vi "LJM logger data file write.vi"(0 "Current Data File In":path, 1 "Write To File":bool, 2 "Currently Writing":bool, 3 "Data File Prefix":string="data", 5 "Working Directory":path, 7 "Log data":string, 9 "Header String":string, 11 "max file size (bytes)":i32=100000000, 15 "Starting #":u32) -> (4 "Current Data File Out":path, 10 "Data File #":u32)   [LabVIEW 2026]
panel:
  out "runtime ms":u32
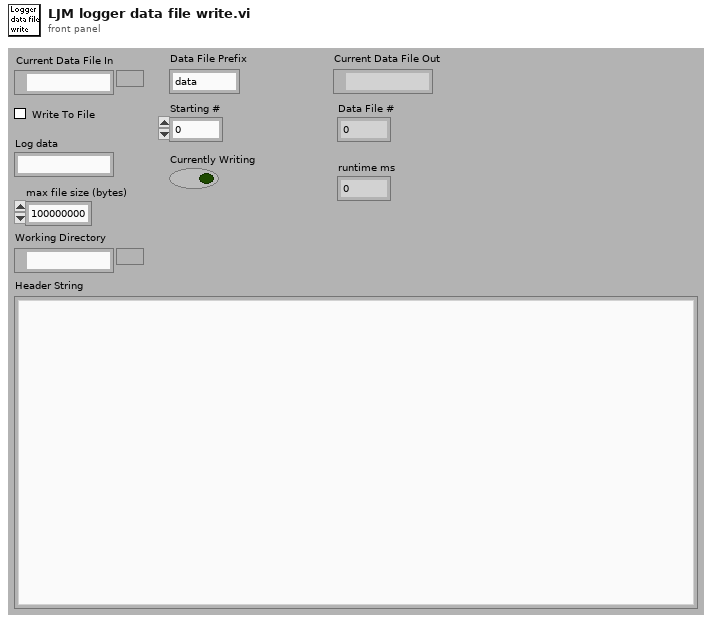
[diagram p1: front panel]
types:
  T1 = enum16{"open", "open or create", "create or replace", "create", "open (read only)"}
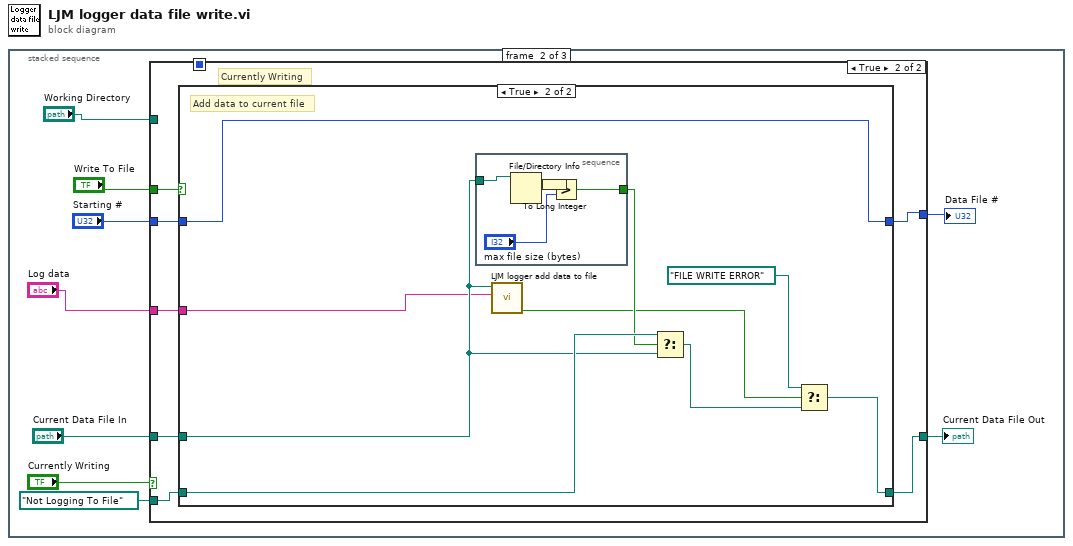
[diagram p0: block diagram]
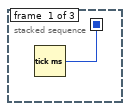
[diagram p2: hidden frame]
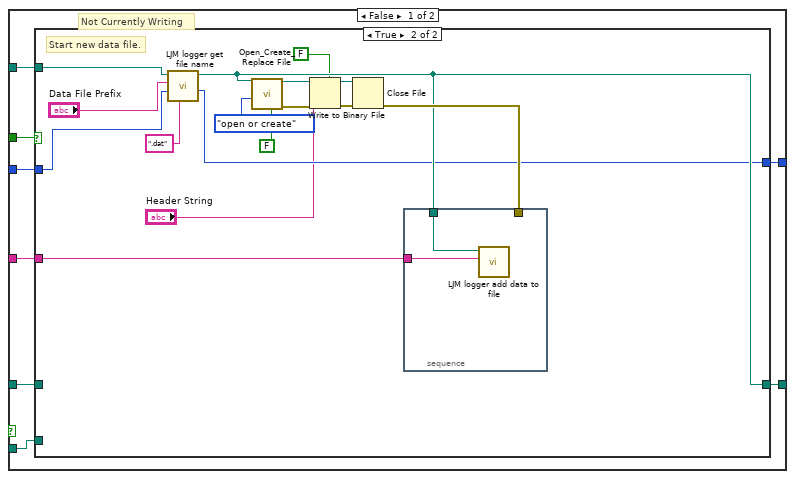
[diagram p3: hidden frame]
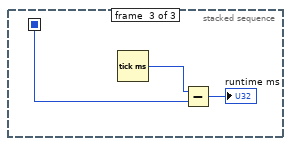
[diagram p6: hidden frame]
diagram:
  n1 = stacked-sequence {
    seq-local: [w1 _ _] -> [_ _ w63]
    frame #0 {
      n2 = Tick Count (ms)() -> (millisecond timer value=w1:u32)
    }
    frame #1 {
      n3 = case shown="True" "Currently Writing" {
        tunnel: "Current Data File In" -> [w18 w45]
        tunnel: "Write To File" -> [w16 w44]
        tunnel: [w17 w42] -> w8
        tunnel: path "Not Logging To File" ("y") -> [w15 w43]
        tunnel: "Starting #" -> [w14 w41]
        tunnel: [w13 w40] -> w5
        tunnel: "Log data" -> [w12 w39]
        tunnel: "Working Directory" -> [w11 _]
        frame False {
          # "Not Currently Writing"
          n4 = case shown="True" w16 {
            tunnel: w18 -> [_ _]
            tunnel: [w20 w28] -> w17
            tunnel: w15 -> [w20 _]
            tunnel: w14 -> [w19 w27]
            tunnel: [w19 w26] -> w13
            tunnel: w12 -> [_ w25]
            tunnel: w11 -> [_ w24]
            frame False {
              # "Do nothing"
            }
            frame True {
              # "Start new data file."
              n5 = call "LJM logger get file name.vi"("Data File Extension"=".dat", "Starting #"=w27, "Data File Prefix"="Data File Prefix", "Working Directory"=w24) -> ("Data File #"=w26:u32, "Data File Path"=w28:path)  [unwired: 6 in]
              n6 = call <vilib>:"Open_Create_Replace File.vi"("advisory dialog? (display:T)"=FALSE, "function (open:0)"=T1."open or create", "file path"=w28) -> ("error out"=w33:errorcluster, "refnum"=w32:refnum<file>)  [unwired: 5 in, 2 out]
              n7 = Write to Binary File(file (use dialog)=w32, data="Header String", error in=w33, 5:FALSE ("prepend array or string size? (T)")) -> (refnum out=w30:refnum<file>, error out=w31:errorcluster)  [unwired: 2 in, 1 out]
              n8 = Close File(refnum=w30, error in=w31) -> (error out=w29:errorcluster)  [unwired: 1 out]
              n9 = stacked-sequence {
                tunnel: w29 -> [_]
                tunnel: w28 -> [w38]
                tunnel: w25 -> [w37]
                frame #0 {
                  n10 = call "LJM logger add data to file.vi"("Data"=w37, "file path"=w38) -> ()  [unwired: 9 in, 1 out]
                }
              }
            }
          }
        }
        frame True {
          # "Currently Writing"
          n11 = case shown="True" w44 {
            tunnel: w45 -> [_ w50]
            tunnel: [w47 w55] -> w42
            tunnel: w43 -> [w47 w53]
            tunnel: w41 -> [w46 w51]
            tunnel: [w46 w51] -> w40
            tunnel: w39 -> [_ w49]
            frame False {
              # "Stop writing to current data file."
            }
            frame True {
              # "Add data to current file"
              n12 = stacked-sequence {
                tunnel: w50 -> [w61]
                tunnel: [w59] -> w52
                frame #0 {
                  n13 = File/Directory Info(path=w61) -> (size=w57:i64)  [unwired: 1 in, 6 out]
                  n14 = To Long Integer(number=w57) -> (32bit integer=w60:i32)
                  n15 = Greater?(x=w60, y="max file size (bytes)") -> (0:w59:bool)
                }
              }
              n16 = call "LJM logger add data to file.vi"("Data"=w49, "file path"=w50) -> ("error"=w48:bool)  [unwired: 9 in]
              n17 = Select(t=w53, s=w52, f=w50) -> (s? t:f=w54:path)
              n18 = Select(t=path "FILE WRITE ERROR", s=w48, f=w54) -> (s? t:f=w55:path)
            }
          }
        }
      }
      "Current Data File Out" <- w8
      "Data File #" <- w5
    }
    frame #2 {
      n19 = Tick Count (ms)() -> (millisecond timer value=w64:u32)
      n20 = Subtract(x=w64, y=w63) -> (x-y=→"runtime ms":u32)
    }
  }
